vi "BRig_Host__Loop_Producer__tcp_System__Data_checkExistence_source.vi"(8 "input_I_arrPath":bool[](array[boolean]), 9 "input_n":i32, 10 "input_arrPath_source":path[](array[path]), 11 "input_arrPath_source_wExpPrefix":path[](array[path])) -> (1 "output_exist_sourceAny":bool[](array[boolean]), 2 "output_exist_source":bool[](array[boolean]), 3 "output_exist_source_wExpPrefix":bool[](array[boolean]))   [LabVIEW 2014]
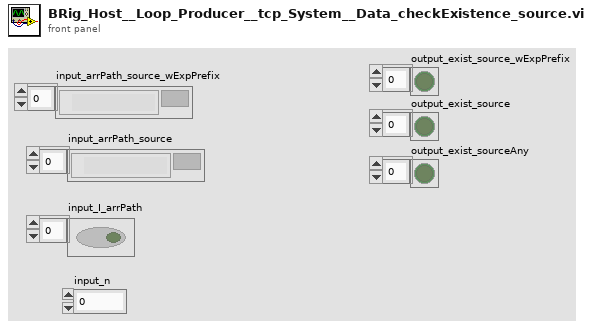
[diagram p1: front panel]
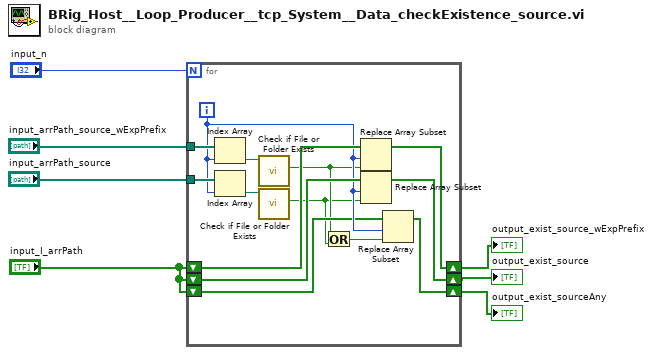
[diagram p0: block diagram]
diagram:
  n1 = for {
    N: "input_n" -> [_]
    tunnel: "input_arrPath_source" -> [w21]
    tunnel: "input_arrPath_source_wExpPrefix" -> [w20]
    shift-right: [w8] -> w3
    shift-left: "input_I_arrPath" -> [w17]
    shift-right: [w9] -> w2
    shift-left: "input_I_arrPath" -> [w16]
    shift-right: [w10] -> w1
    shift-left: "input_I_arrPath" -> [w14]
    i -> [w15]
    n2 = Index Array(array=w20, index=w15) -> (element=w19:path)
    n3 = Index Array(array=w21, index=w15) -> (element=w18:path)
    n4 = call <vilib>:"Check if File or Folder Exists.vi"("path"=w19) -> ("file or folder exists?"=w13:bool)  [unwired: 8 in, 2 out]
    n5 = call <vilib>:"Check if File or Folder Exists.vi"("path"=w18) -> ("file or folder exists?"=w12:bool)  [unwired: 8 in, 2 out]
    n6 = Or(x=w13, y=w12) -> (x .or. y?=w11:bool)
    n7 = Replace Array Subset(array=w17, new element=w13, index=w15) -> (w8:bool[])
    n8 = Replace Array Subset(array=w16, new element=w12, index=w15) -> (w9:bool[])
    n9 = Replace Array Subset(array=w14, new element=w11, index=w15) -> (w10:bool[])
  }
  "output_exist_source_wExpPrefix" <- w3
  "output_exist_source" <- w2
  "output_exist_sourceAny" <- w1
